vi "Handle File Patterns.vi"(9 "Search Class(*.lvclass)":bool, 10 "Search Librerieries(*.lvlib)":bool=TRUE, 11 "pattern":string[](array[string])) -> (3 "Pattern out":string[](array[string]))   [LabVIEW 2019, in "SimpleDependencyInspector.lvlib"]
uses:
  SimpleDependencyInspector.lvlib
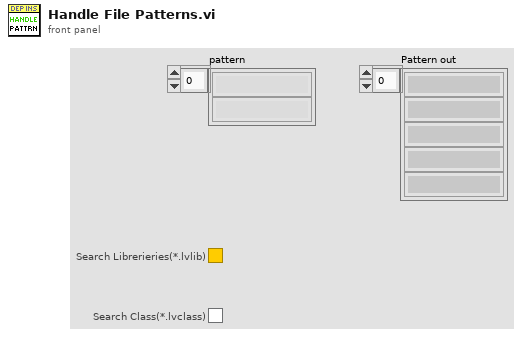
[diagram p1: front panel]
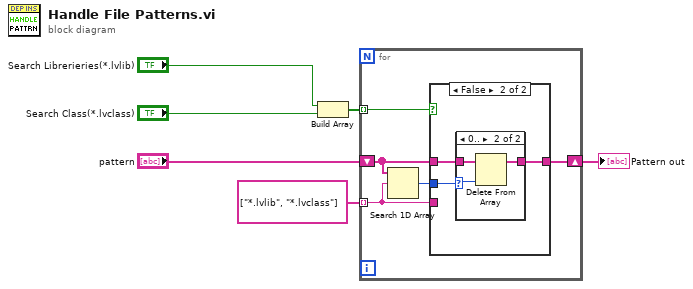
[diagram p0: block diagram]
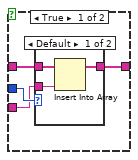
[diagram p2: hidden frame]
diagram:
  n1 = Build Array("Search Librerieries(*.lvlib)", "Search Class(*.lvclass)") -> (w3:bool[])
  n2 = for {
    tunnel: w3 -> [w11] mode=indexing
    tunnel: string[] ["*.lvlib", "*.lvclass"] ("pattern") -> [w8] mode=indexing
    shift-right: [w7] -> w4
    shift-left: "pattern" -> [w10]
    n3 = Search 1D Array(1D array=w10, element=w8) -> (index of element=w9:i32)  [unwired: 1 in]
    n4 = case shown="False" w11 {
      tunnel: w10 -> [w14 w21]
      tunnel: [w13 w20] -> w7
      tunnel: w9 -> [w15 w22]
      tunnel: w8 -> [w12 _]
      frame True {
        n5 = case shown="Default" w15 {
          tunnel: w14 -> [w18 w19]
          tunnel: [w17 w19] -> w13
          tunnel: w12 -> [w16 _]
          frame Default {
            n6 = Insert Into Array(array=w18, new element=w16) -> (w17:string[])  [unwired: 1 in]
          }
          frame 0.. {
          }
        }
      }
      frame False {
        n7 = case shown="0.." w22 {
          selector: w22 -> [_ w24]
          tunnel: w21 -> [w23 w26]
          tunnel: [w23 w25] -> w20
          frame Default {
          }
          frame 0.. {
            n8 = Delete From Array(array=w26, index=w24) -> (array with subset deleted=w25:string[])  [unwired: 1 in, 1 out]
          }
        }
      }
    }
  }
  "Pattern out" <- w4
